vi "UpdateNv.vi"(0 "Pump_1AI_1DO_2DI in":refnum<class "NeedleValve.lvclass">, 11 "error in (no error)":errorcluster, 13 "modbus":refnum<class "Modbus Master.lvclass">) -> (4 "Pump_1AI_1DO_2DI out":refnum<class "NeedleValve.lvclass">, 14 "Connected":bool, 15 "error out":errorcluster)   [LabVIEW 2019, in "NeedleValve.lvclass"]
uses:
  NeedleValve.lvclass
  C:/Users/ANENKOV_V1/Desktop/SRC_H400/src/Proccess_class/Proccess.lvclass
  C:/Users/ANENKOV_V1/Desktop/SRC_H400/src/Device_class/Device.lvclass
  <vilib>/NI/Modbus Library/API/Master/Modbus Master.lvclass
  NeedleValve.lvclass/NeedleValve.ctl
  Proccess_class/Proccess.lvclass/Proccess.ctl
  modbus engine custom/MB_MODULE_class/MB_MODULE.lvclass/MB_MODULE.ctl
  Proccess_class/GetNames.vi
  Proccess_class/GetLogger.vi
  private/SendToDb.vi/ddaf1088-39ed-46bc-a000-2f82a45c55df.vi
  Device_class/ErrorToDb.vi/d458cff9-8e45-4544-91af-cfa5b3c8a69c.vi
  Device_class/Device.lvclass
  modbus engine custom/MB_ENGINE_class/MB_ENGINE.lvclass
  C:/Users/ANENKOV_V1/Desktop/SRC_H400/src/modbus engine custom/MB_MODULE_class/MB_MODULE.lvclass
  Logger_class/WriteEvent.vi
  modbus engine custom/MB_MODULE_class/MB_MODULE.lvclass
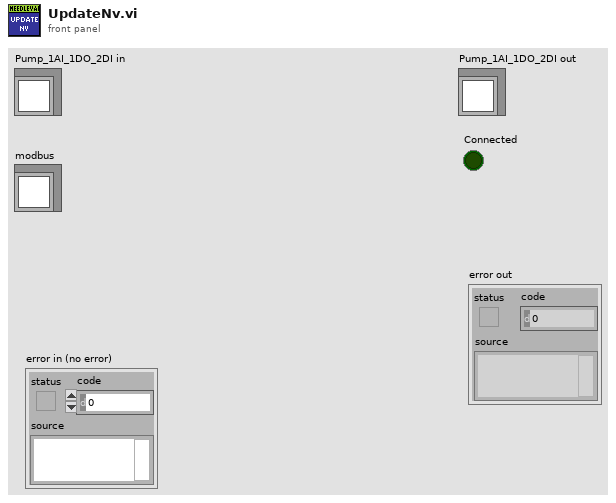
[diagram p1: front panel]
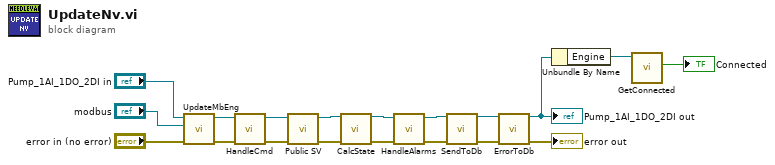
[diagram p0: block diagram]
diagram:
  n1 = call "UpdateMbEng.vi"("error in (no error)"="error in (no error)", "modbus"="modbus", "NeedleValve in"="Pump_1AI_1DO_2DI in") -> ("error out"=w17:errorcluster, "NeedleValve out"=w16:refnum<class "NeedleValve.lvclass">)  [unwired: 7 in]
  n2 = call "HandleCmd.vi"("error in (no error)"=w17, "NeedleValve in"=w16) -> ("error out"=w14:errorcluster, "NeedleValve out"=w15:refnum<class "NeedleValve.lvclass">)  [unwired: 8 in]
  n3 = call "Public SV.vi"("error in (no error)"=w14, "NeedleValve in"=w15) -> ("error out"=w3:errorcluster, "NeedleValve out"=w4:refnum<class "NeedleValve.lvclass">)  [unwired: 8 in]
  n4 = call "CalcState.vi"("reference in"=w4, "error in (no error)"=w3) -> ("reference out"=w2:refnum<class "NeedleValve.lvclass">, "error out"=w1:errorcluster)  [unwired: 12 in]
  n5 = call "HandleAlarms.vi"("error in (no error)"=w1, "NeedleValve in"=w2) -> ("error out"=w6:errorcluster, "NeedleValve out"=w5:refnum<class "NeedleValve.lvclass">)  [unwired: 8 in]
  n6 = call "SendToDb.vi"("reference in"=w5, "error in (no error)"=w6) -> ("reference out"=w13:refnum<class "NeedleValve.lvclass">, "error out"=w12:errorcluster)  [unwired: 12 in]
  n7 = call "ErrorToDb.vi"("reference in"=w13, "error in (no error)"=w12) -> ("reference out"=w10:refnum<class "NeedleValve.lvclass">, "error out"=→"error out":errorcluster)  [unwired: 12 in]
  "Pump_1AI_1DO_2DI out" <- w10
  n8 = Unbundle By Name(w10) -> ("Engine"=w8:refnum<class "MB_ENGINE.lvclass">)
  n9 = call "GetConnected.vi"("MB_MODULE in"=w8) -> ("Connected"=→"Connected":bool)  [unwired: 10 in]
